vi "Method One Numeric Argument.vi"(8 "error in (no error)":errorcluster, 10 "Numeric":dbl, 11 "Test Interface Mock In":refnum<class "Test Interface Mock.lvclass">) -> (0 "error out":errorcluster, 3 "Test Interface Mock Out":refnum<class "Test Interface Mock.lvclass">)   [LabVIEW 2020, in "Test Interface Mock.lvclass"]
uses:
  Test Interface Mock.lvclass
  C:/git/astemes-lmock/sandbox/Mock/Mock.lvclass
  Mock/Mock.lvclass
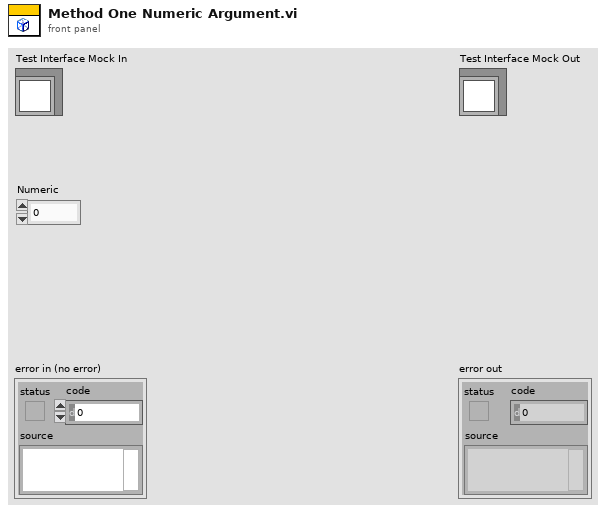
[diagram p1: front panel]
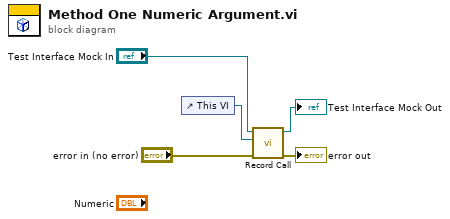
[diagram p0: block diagram]
diagram:
  n1 = control-ref of="This VI"() -> (w5:refnum<vi>)
  n2 = call "Record Call.vi"("error in (no error)"="error in (no error)", "This VI"=w5, "Mock In"="Test Interface Mock In") -> ("error out"=→"error out":errorcluster, "Mock Out"=→"Test Interface Mock Out":refnum<class "Test Interface Mock.lvclass">)  [unwired: 7 in]
